vi "CRYCalc best fit of average.vi"(7 "Step Setup VI No":i32, 9 "rank number(best curve)":i32, 11 "Data in":T1 {"Z data" items=["dB", "Lin"]; "X data" items=["dB", "Lin"]; "Y data" items=["dB", "Lin"]; "Z dB ref" format="%.1f"; "Z axis" items=["Log", "Lin"]; "X dB ref" format="%.1f"; "X axis" items=["Log", "Lin"]; "Y axis" items=["Log", "Lin"]; "Y dB ref" format="%.1f"; "Curve"."z" format="%.2f"; "Curve"."y" format="%.2f"; "Curve"."x" format="%.2f"}) -> (3 "Best Fit Out":T1 {"Z data" items=["dB", "Lin"]; "X data" items=["dB", "Lin"]; "Y data" items=["dB", "Lin"]; "Z dB ref" format="%.1f"; "Z axis" items=["Log", "Lin"]; "X dB ref" format="%.1f"; "X axis" items=["Log", "Lin"]; "Y axis" items=["Log", "Lin"]; "Y dB ref" format="%.1f"; "Curve"."z" format="%.2f"; "Curve"."y" format="%.2f"; "Curve"."x" format="%.2f"})   [LabVIEW 2013]
uses:
  Typedef Control/CRYData Cluster Array.ctl
  Typedef Control/CRYData Cluster.ctl
  <vilib>/Analysis/NI_AALBase.lvlib
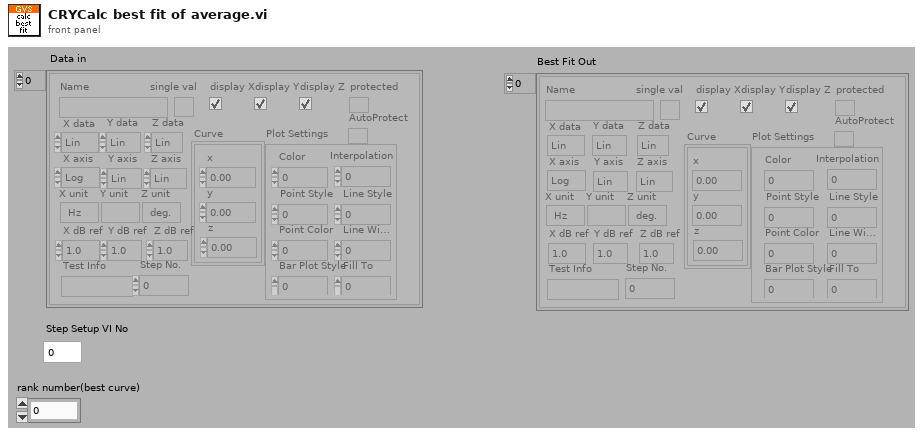
[diagram p1: front panel]
types:
  T1 = typedef "CRYData Cluster Array.ctl" = T2[]
  T2 = typedef "CRYData Cluster.ctl" = cluster{"Name":string, "Curve":cluster{"x":dbl, "y":dbl, "z":dbl}[], "X data":u16, "Y data":u16, "Z data":u16, "X axis":u16, "Y axis":u16, "Z axis":u16, "X unit":string, "Y unit":string, "Z unit":string, "X dB ref":dbl, "Y dB ref":dbl, "Z dB ref":dbl, "single val":bool, "protected":bool, "display X":bool, "display Y":bool, "display Z":bool, "Test Info":string, "Step No.":i32, "Plot Settings":cluster{"Color":u32, "Interpolation":u8, "Point Style":u8, "Line Style":u8, "Point Color":u32, "Line Width":u8, "Bar Plot Style":u8, "Fill To":i16}, "AutoProtect":bool}
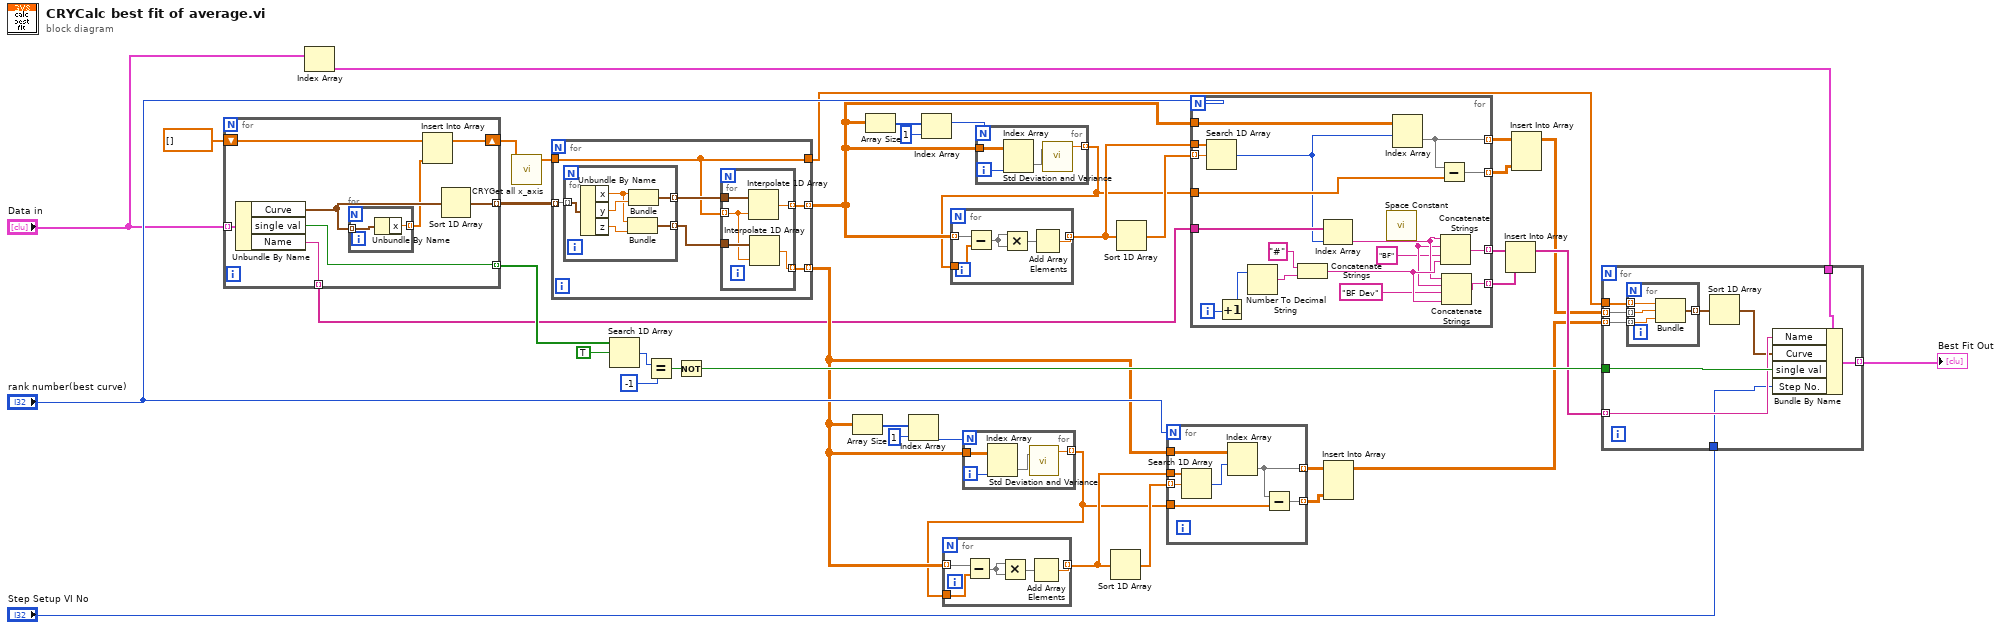
[diagram p0: block diagram]
diagram:
  n1 = for {
    tunnel: [w41] -> w33 mode=indexing
    tunnel: "Data in" -> [w43] mode=indexing
    shift-right: [w46] -> w14
    shift-left: dbl[] [] ("x_Array") -> [w45]
    tunnel: [w44] -> w35 mode=indexing
    tunnel: [w42] -> w2 mode=indexing
    n2 = Unbundle By Name(w43) -> ("Curve"=w48:cluster{"x":dbl, "y":dbl, "z":dbl}[], "single val"=w44:bool, "Name"=w42:string)
    n3 = for {
      tunnel: w48 -> [w49] mode=indexing
      tunnel: [w50] -> w47 mode=indexing
      n4 = Unbundle By Name(w49) -> ("x"=w50:dbl)
    }
    n5 = Insert Into Array(array=w45, new element=w47) -> (w46:dbl[])  [unwired: 1 in]
    n6 = Sort 1D Array(array=w48) -> (sorted array=w41:cluster{"x":dbl, "y":dbl, "z":dbl}[])
  }
  n7 = Index Array(array="Data in") -> (element=w37:T2)  [unwired: 1 in]
  n8 = call "CRYGet all x_axis.vi"("x_Array in"=w14) -> ("X_axis out"=w32:dbl[])  [unwired: 1 in, 9 out]
  n9 = for {
    tunnel: w33 -> [w52] mode=indexing
    tunnel: [w56] -> w17 mode=indexing
    tunnel: w32 -> [w51]
    tunnel: [w51] -> w36
    tunnel: [w53] -> w6 mode=indexing
    n10 = for {
      tunnel: [w61] -> w55 mode=indexing
      tunnel: w52 -> [w60] mode=indexing
      tunnel: [w57] -> w54 mode=indexing
      n11 = Unbundle By Name(w60) -> ("x"=w58:dbl, "y"=w62:dbl, "z"=w59:dbl)
      n12 = Bundle("x"=w58, "z"=w59) -> (w57:cluster{"x":dbl, "z":dbl})  [unwired: 1 out]
      n13 = Bundle("x"=w58, "y"=w62) -> (w61:cluster{"x":dbl, "y":dbl})  [unwired: 1 out]
    }
    n14 = for {
      tunnel: [w67] -> w56 mode=indexing
      tunnel: w55 -> [w66]
      tunnel: w51 -> [w64] mode=indexing
      tunnel: w54 -> [w65]
      tunnel: [w63] -> w53 mode=indexing
      n15 = Interpolate 1D Array(1:w64, 2:w66) -> (0:w67:dbl)
      n16 = Interpolate 1D Array(1:w64, 2:w65) -> (0:w63:dbl)
    }
  }
  n17 = Search 1D Array(1D array=w35, element=TRUE) -> (index of element=w30:i32)  [unwired: 1 out]
  n18 = Equal?(x=w30, y=-1) -> (x = y?=w28:bool)
  n19 = Not(x=w28) -> (.not. x?=w27:bool)
  n20 = Array Size(array=w6) -> (size(s)=w11:i32[])
  n21 = Array Size(array=w17) -> (size(s)=w22:i32[])
  n22 = Index Array(array=w11, index=1) -> (element=w10:i32)
  n23 = Index Array(array=w22, index=1) -> (element=w23:i32)
  n24 = for {
    N: w10 -> [_]
    tunnel: w6 -> [w71]
    tunnel: [w69] -> w3 mode=indexing
    i -> [w68]
    n25 = Index Array(array=w71, index (col)=w68) -> (element=w70:dbl[])  [unwired: 1 in]
    n26 = call <vilib>:"Std Deviation and Variance.vi"("X"=w70) -> ("mean"=w69:dbl)  [unwired: 1 in, 2 out]
  }
  n27 = for {
    tunnel: w6 -> [w72] mode=indexing
    tunnel: w3 -> [w75]
    tunnel: [w76] -> w8 mode=indexing
    n28 = Subtract(x=w72, y=w75) -> (x-y=w73:dbl[])
    n29 = Multiply(x=w73, y=w73) -> (x*y=w74:dbl[])
    n30 = Add Array Elements(numeric array=w74) -> (sum=w76:dbl)
  }
  n31 = for {
    N: w23 -> [_]
    tunnel: w17 -> [w80]
    tunnel: [w78] -> w4 mode=indexing
    i -> [w77]
    n32 = Index Array(array=w80, index (col)=w77) -> (element=w79:dbl[])  [unwired: 1 in]
    n33 = call <vilib>:"Std Deviation and Variance.vi"("X"=w79) -> ("mean"=w78:dbl)  [unwired: 1 in, 2 out]
  }
  n34 = for {
    tunnel: w17 -> [w81] mode=indexing
    tunnel: w4 -> [w84]
    tunnel: [w85] -> w25 mode=indexing
    n35 = Subtract(x=w81, y=w84) -> (x-y=w82:dbl[])
    n36 = Multiply(x=w82, y=w82) -> (x*y=w83:dbl[])
    n37 = Add Array Elements(numeric array=w83) -> (sum=w85:dbl)
  }
  n38 = Sort 1D Array(array=w8) -> (sorted array=w9:dbl[])
  n39 = Sort 1D Array(array=w25) -> (sorted array=w24:dbl[])
  n40 = for {
    N: "rank number(best curve)" -> [_]
    tunnel: w9 -> [w91] mode=indexing
    tunnel: w6 -> [w90]
    tunnel: w8 -> [w92]
    tunnel: [w87] -> w12 mode=indexing
    tunnel: [w88] -> w13 mode=indexing
    tunnel: w3 -> [w86]
    n41 = Search 1D Array(1D array=w92, element=w91) -> (index of element=w89:i32)  [unwired: 1 out]
    n42 = Index Array(array=w90, index (row)=w89) -> (element=w87:dbl[])  [unwired: 1 in]
    n43 = Subtract(x=w87, y=w86) -> (x-y=w88:dbl[])
  }
  n44 = for {
    N: "rank number(best curve)" -> [_]
    tunnel: w24 -> [w110] mode=indexing
    tunnel: w17 -> [w109]
    tunnel: w25 -> [w111]
    tunnel: [w104] -> w21 mode=indexing
    tunnel: [w105] -> w20 mode=indexing
    tunnel: w2 -> [w108]
    tunnel: [w107] -> w18 mode=indexing
    tunnel: [w106] -> w19 mode=indexing
    tunnel: w4 -> [w103]
    i -> [w101]
    n45 = Search 1D Array(1D array=w111, element=w110) -> (index of element=w102:i32)  [unwired: 1 out]
    n46 = Increment(x=w101) -> (x+1=w100:i32)
    n47 = Number To Decimal String(number=w100) -> (decimal integer string=w99:string)  [unwired: 1 out]
    n48 = Concatenate Strings("#" ("string"), w99) -> (w97:string)
    n49 = Index Array(array=w108, index=w102) -> (element=w96:string)
    n50 = call <vilib>:"Space Constant.vi"() -> ("String"=w95:string)
    n51 = Index Array(array=w109, index (row)=w102) -> (element=w104:dbl[])  [unwired: 1 in]
    n52 = Subtract(x=w104, y=w103) -> (x-y=w105:dbl[])
    n53 = Concatenate Strings(w96, w95, "BF", w97) -> (w106:string)
    n54 = Concatenate Strings(w96, w95, "BF Dev", w97) -> (w107:string)
  }
  n55 = Insert Into Array(array=w12, new element=w13) -> (w5:dbl[][])  [unwired: 2 in]
  n56 = Insert Into Array(array=w19, new element=w18) -> (w16:string[])  [unwired: 1 in]
  n57 = Insert Into Array(array=w21, new element=w20) -> (w15:dbl[][])  [unwired: 2 in]
  n58 = for {
    tunnel: w36 -> [w121]
    tunnel: w5 -> [w120] mode=indexing
    tunnel: w27 -> [w119]
    tunnel: [w117] -> w40 mode=indexing
    tunnel: w16 -> [w116] mode=indexing
    tunnel: w15 -> [w115] mode=indexing
    tunnel: w37 -> [w114]
    tunnel: "Step Setup VI No" -> [w112]
    n59 = for {
      tunnel: w115 -> [w124] mode=indexing
      tunnel: [w125] -> w118 mode=indexing
      tunnel: w121 -> [w123] mode=indexing
      tunnel: w120 -> [w122] mode=indexing
      n60 = Bundle("x"=w123, w124, w122) -> (w125:cluster{"x":dbl, dbl, dbl})  [unwired: 1 out]
    }
    n61 = Sort 1D Array(array=w118) -> (sorted array=w113:cluster{"x":dbl, dbl, dbl}[])
    n62 = Bundle By Name(cluster=w114, "Name"=w116, "Curve"=w113, "single val"=w119, "Step No."=w112) -> (w117:T2)
  }
  "Best Fit Out" <- w40
